vi "XYStage.KIM101.MoveAbsoluteByAxis (counts).vi"(8 "error in (no error)":errorcluster, 9 "Position (counts)":i32, 10 "Axis":T1, 11 "XYStage.KIM101 in":refnum<class "XYStage.KIM101.lvclass">) -> (0 "error out":errorcluster, 3 "XYStage.KIM101 out":refnum<class "XYStage.KIM101.lvclass">)   [LabVIEW 2019, in "XYStage.KIM101.lvclass"]
uses:
  XYStage.KIM101.lvclass
  XYStage/Typedefs/XYStage.Axis--Enum.ctl
  E:/UPWORK/NTU-APR-LAB/photonics-measurements-tool-labview/project/data/Thorlabs.MotionControl.KCube.InertialMotorCLI.dll
  data/Thorlabs.MotionControl.KCube.InertialMotorCLI.dll
  XYStage/XYStage.lvclass
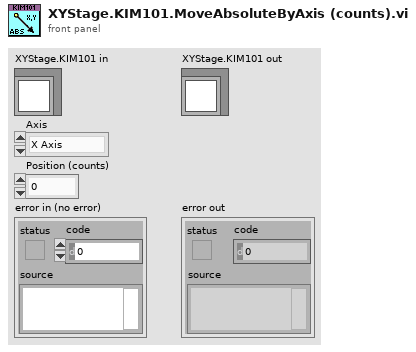
[diagram p1: front panel]
types:
  T1 = typedef "XYStage.lvclass/XYStage.Axis--Enum.ctl" = enum16{"X Axis", "Y Axis", "Undefined"}
  T2 = typedef "XYStage.KIM101.lvclass/Resource--Cluster.ctl" = cluster{"KCubeInertialMotorControl":refnum<k24>, "Device":refnum<k24>, "X Axis Channel":i32, "Y Axis Channel":i32}
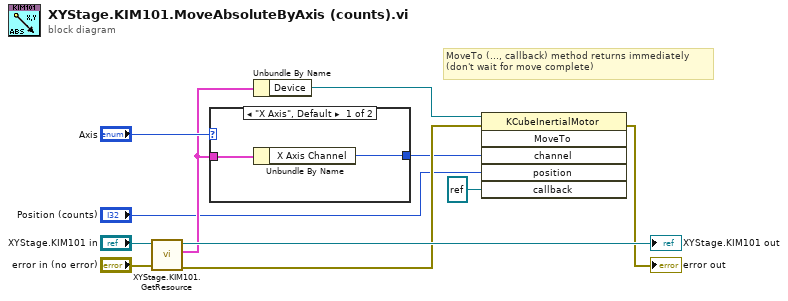
[diagram p0: block diagram]
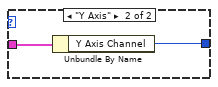
[diagram p2: hidden frame]
diagram:
  # "MoveTo (..., callback) method returns immediately\n(don't wait for move complete)"
  n1 = call "XYStage.KIM101.GetResource.vi"("error in (no error)"="error in (no error)", "XYStage.KIM101 in"="XYStage.KIM101 in") -> ("error out"=w6:errorcluster, "Resource"=w4:T2, "XYStage.KIM101 out"=→"XYStage.KIM101 out":refnum<class "XYStage.KIM101.lvclass">)  [unwired: 7 in]
  n2 = case shown="\"X Axis\", Default" "Axis" {
    tunnel: w4 -> [w13 w15]
    tunnel: [w12 w14] -> w3
    frame "X Axis", Default {
      n3 = Unbundle By Name(w13) -> ("X Axis Channel"=w12:i32)
    }
    frame "Y Axis" {
      n4 = Unbundle By Name(w15) -> ("Y Axis Channel"=w14:i32)
    }
  }
  n5 = Unbundle By Name(w4) -> ("Device"=w8:refnum<k24>)
  n6 = invoke class="KCubeInertialMotor" method="MoveTo"(reference=w8, error in=w6, "channel"=w3, "position"="Position (counts)", "callback"=refnum<k24> refnum) -> (error out=→"error out":errorcluster)  [unwired: 1 in, 5 out]
